vi "未命名 1.vi"   [LabVIEW 2014]
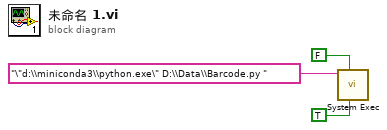
[diagram p0: block diagram]
diagram:
  n1 = call <vilib>:"System Exec.vi"("run minimized? (F)"=TRUE, "wait until completion? (T)"=FALSE, "command line"="\"d:\\miniconda3\\python.exe\" D:\\Data\\Barcode.py ") -> ()  [unwired: 5 in, 4 out]
